vi "Init UI.vi"(8 "error in (no error)":errorcluster, 11 "HistorianCharting in":refnum<class "HistorianCharting.lvclass">) -> (0 "error out":errorcluster, 3 "HistorianCharting out":refnum<class "HistorianCharting.lvclass">)   [LabVIEW 2020, in "VolatusGUIElements.lvlib" / "HistorianCharting.lvclass"]
uses:
  HistorianCharting.lvclass
  HistorianCharting.lvclass/HistorianCharting.ctl
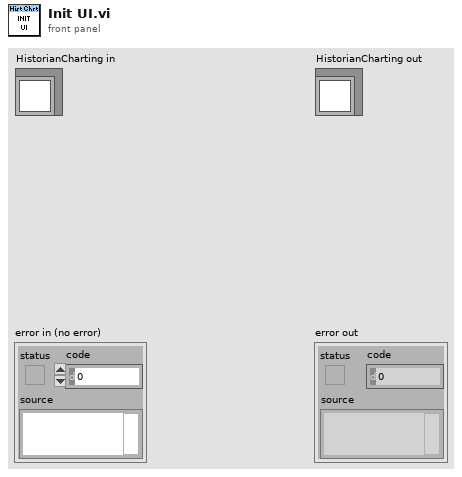
[diagram p1: front panel]
types:
  T1 = cluster{"Channel":string, "Value":dbl, "Color":u32, "Scale":bool, "Visible":bool}[]
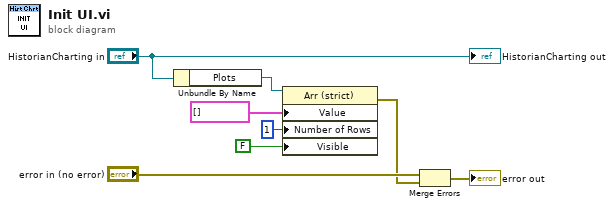
[diagram p0: block diagram]
diagram:
  n1 = Unbundle By Name("HistorianCharting in") -> ("Plots"=w6:refnum<vi>)
  n2 = property class="Arr (strict)"(reference=w6, "Value"=T1 [], "Number of Rows"=u32 1, "Visible"=FALSE) -> (error out=w1:errorcluster)  [unwired: 1 in, 1 out]
  n3 = Merge Errors("error in (no error)", w1) -> (→"error out":errorcluster)
  "HistorianCharting out" <- "HistorianCharting in"
